vi "Parallel For Loop Reduction.vi"() -> ()   [LabVIEW 2023]
doc: "This VI contains a parallel For Loop that computes the sum reduction of an array using shift registers."
panel:
  in  "Array":dbl[](array[numeric])=array[10000 elements]
  in  "Tolerance":dbl=1e-08
  out "Sums Match":bool
  # "Overview: Demonstrates the use of a Parallel For Loop to perform a scalar reduction operation in parallel.\nInstructions:\nRun the VI. The sum of the array is calculated both as a reduction in a Parallel For Loop, and with the Add Array Elements function. See the block diagram for more information."
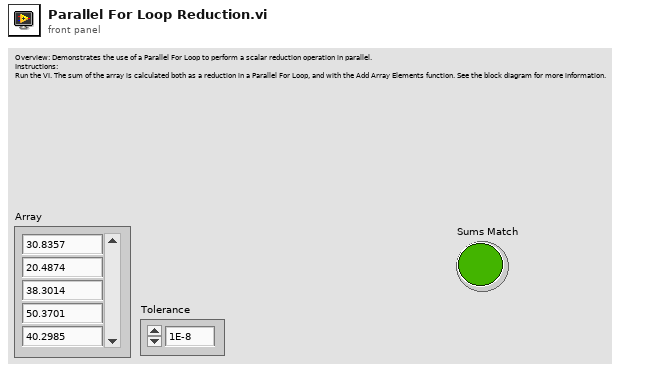
[diagram p1: front panel]
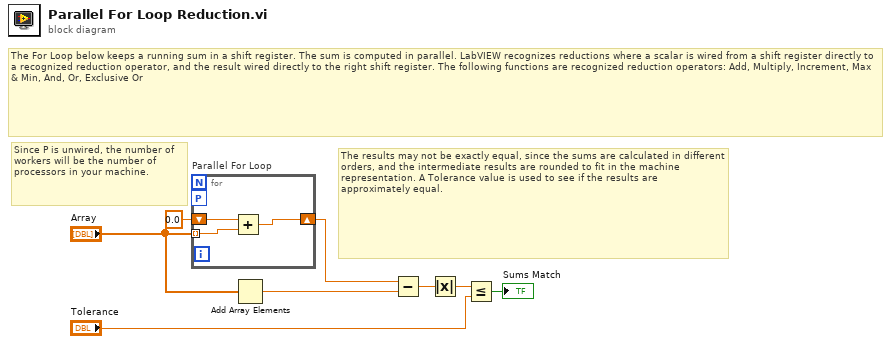
[diagram p0: block diagram]
diagram:
  # "The results may not be exactly equal, since the sums are calculated in different orders, and the intermediate results are rounded to fit in the machine representation. A Tolerance value is used to see if the results are approximately equal."
  # "Since P is unwired, the number of workers will be the number of processors in your machine."
  # "The For Loop below keeps a running sum in a shift register. The sum is computed in parallel. LabVIEW recognizes reductions where a scalar is wired from a shift register directly to a recognized reduction operator, and the result wired directly to the right shift register. The following functions are recognized reduction operators: Add, Multiply, Increment, Max & Min, And, Or, Exclusive Or"
  n1 = for "Parallel For Loop" {
    shift-right: [w9] -> w7
    shift-left: 0.0 ("element") -> [w11]
    tunnel: "Array" -> [w10] mode=indexing
    workers-P: _ -> [_]
    n2 = Add(x=w11, y=w10) -> (x+y=w9:dbl)
  }
  n3 = Add Array Elements(numeric array="Array") -> (sum=w6:dbl)
  n4 = Subtract(x=w7, y=w6) -> (x-y=w5:dbl)
  n5 = Absolute Value(x=w5) -> (abs(x)=w4:dbl)
  n6 = Less Or Equal?(x=w4, y="Tolerance") -> (x <= y?=→"Sums Match":bool)
